vi "OAT Get Masks for Synthesis.vi"(8 "orders to extract":cluster{"orders to extract":dbl[]}[](array[cluster]), 10 "order sequence":dbl[](array[numeric]), 11 "mask":bool[][][](array[boolean])) -> (0 "order list":string[](array[string]), 3 "synthesis mask":bool[][][](array[boolean]))   [LabVIEW 2017, in "SoundVib_Gabor.lvlib"]
uses:
  <vilib>/addons/Sound and Vibration/Order Analysis/Gabor Order Tracking/SoundVib_Gabor.lvlib
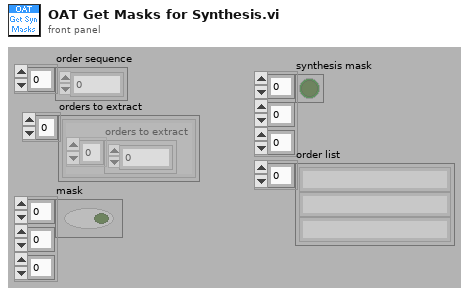
[diagram p1: front panel]
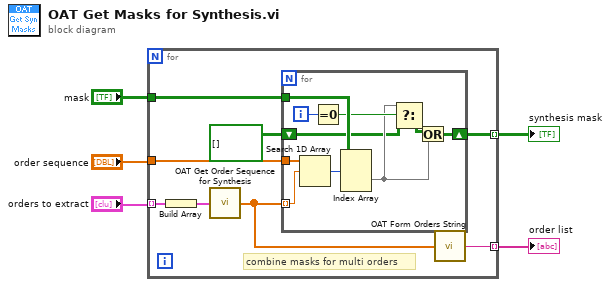
[diagram p0: block diagram]
diagram:
  n1 = for {
    tunnel: "orders to extract" -> [w8] mode=indexing
    tunnel: "order sequence" -> [w13]
    tunnel: "mask" -> [w11]
    tunnel: [w10] -> w2 mode=indexing
    tunnel: [w9] -> w1 mode=indexing
    # "combine masks for multi orders"
    n2 = Build Array(w8) -> (w6:cluster{"orders to extract":dbl[]}[])
    n3 = call <vilib>:"OAT Get Order Sequence for Synthesis.vi"("orders to extract"=w6) -> ("order sequence"=w7:dbl[])  [unwired: 4 in]
    n4 = for {
      tunnel: w7 -> [w14] mode=indexing
      tunnel: w13 -> [w23]
      tunnel: w11 -> [w22]
      shift-right: [w15] -> w10
      shift-left: bool[][] [] ("mask array") -> [w17]
      i -> [w20]
      n5 = Search 1D Array(1D array=w23, element=w14) -> (index of element=w21:i32)  [unwired: 1 in]
      n6 = Equal To 0?(x=w20) -> (x = 0?=w19:bool)
      n7 = Index Array(array=w22, index (dim 0)=w21) -> (element=w18:bool[][])  [unwired: 2 in]
      n8 = Select(t=w18, s=w19, f=w17) -> (s? t:f=w16:bool[][])
      n9 = Or(x=w16, y=w18) -> (x .or. y?=w15:bool[][])
    }
    n10 = call <vilib>:"OAT Form Orders String.vi"("orders to extract in"=w7) -> ("orders to extract out"=w9:string)
  }
  "synthesis mask" <- w2
  "order list" <- w1
